vi "Open.vi"(7 "I2C Channel":u8, 8 "Error In":errorcluster, 10 "I2C Slave Address (0x1D)":u8=29 format="%.0x", 11 "LINX Ref":T1) -> (0 "Error Out":errorcluster, 3 "LINX Resource":T1)   [LabVIEW 2014, in "LMH-LINX.lvlib" / "MMA8452.lvlib"]
doc: "Open the I2C master and initialize the MMA8452 accelerometer.\n\nIf the LINX device has more than one I2C master the logical first I2C master is channel 0, the next is channel 1, etc."
uses:
  <vilib>/MakerHub/LINX/Public/Sensors/Accelerometer/MMA8452/MMA8452.lvlib
  <vilib>/MakerHub/LINX/Private/Type Defs/LINX Ref.ctl
  <vilib>/MakerHub/LINX/Private/Type Defs/Platform.ctl
  <vilib>/MakerHub/LINX/Private/Type Defs/Interface.ctl
  <vilib>/MakerHub/LINX/Private/Device/Type Defs/LINX Device Config.ctl
  <vilib>/MakerHub/LINX/Private/Device/Type Defs/TCP Config.ctl
  <vilib>/MakerHub/LINX/Private/Device/Type Defs/Channels.ctl
  <vilib>/MakerHub/LINX/Private/Type Defs/Peripherals/I2C/EOF.ctl
  <vilib>/MakerHub/LINX/Private/Local IO/LinxI2cWrite.vi
  <vilib>/MakerHub/LINX/Public/Utilities/Check Channel.vi
  <vilib>/MakerHub/LINX/Private/Utilties/Generate Error.vi
  <vilib>/MakerHub/LINX/LMH-LINX.lvlib
  <vilib>/MakerHub/LINX/Private/Device/Device.lvlib
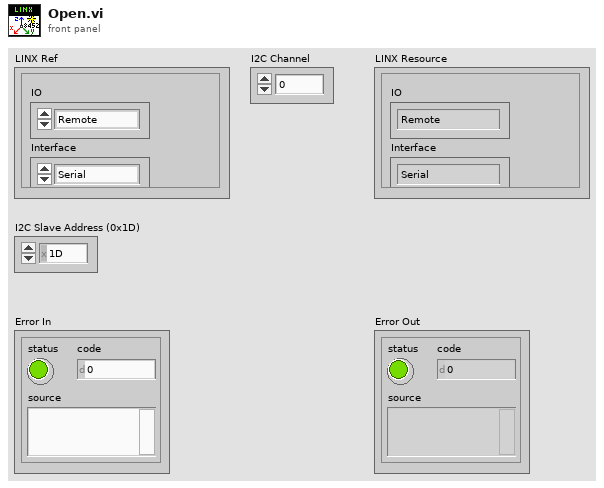
[diagram p1: front panel]
types:
  T1 = typedef "LMH-LINX.lvlib/LINX Ref.ctl" = cluster{"IO":T2, "Interface":T3, "LINX Device Config":T4}
  T2 = typedef "LMH-LINX.lvlib/Platform.ctl" = enum16{"Remote", "Local"}
  T3 = typedef "LMH-LINX.lvlib/Interface.ctl" = enum16{"Serial", "TCP"}
  T4 = typedef "LMH-LINX.lvlib/Device.lvlib/LINX Device Config.ctl" = cluster{"Interface":T3, "COM Port":refnum<visa-resource-name>, "TCP Configuration":T5, "Device Family":u8, "Device ID":u8, "Device Name":string, "TCP Ref":refnum<k5>, "Channels":T6}
  T5 = typedef "LMH-LINX.lvlib/Device.lvlib/TCP Config.ctl" = cluster{"IP Address":string, "Port":u16}
  T6 = typedef "LMH-LINX.lvlib/Channels.ctl" = cluster{"DI":u8[], "DO":u8[], "AI":u8[], "AO":u8[], "PWM":u8[], "QE":u8[], "UART":u8[], "I2C 2":u8[], "SPI":u8[], "CAN":u8[], "Servo":u8[], "AI Ref (V)":dbl, "AI Resolution (Bits)":u8, "AO Ref (V)":dbl, "AO Resolution (Bits)":u8}
  T7 = typedef "LMH-LINX.lvlib/EOF.ctl" = enum8{"Stop", "Restart", "Restart No Stop", "No Stop"}
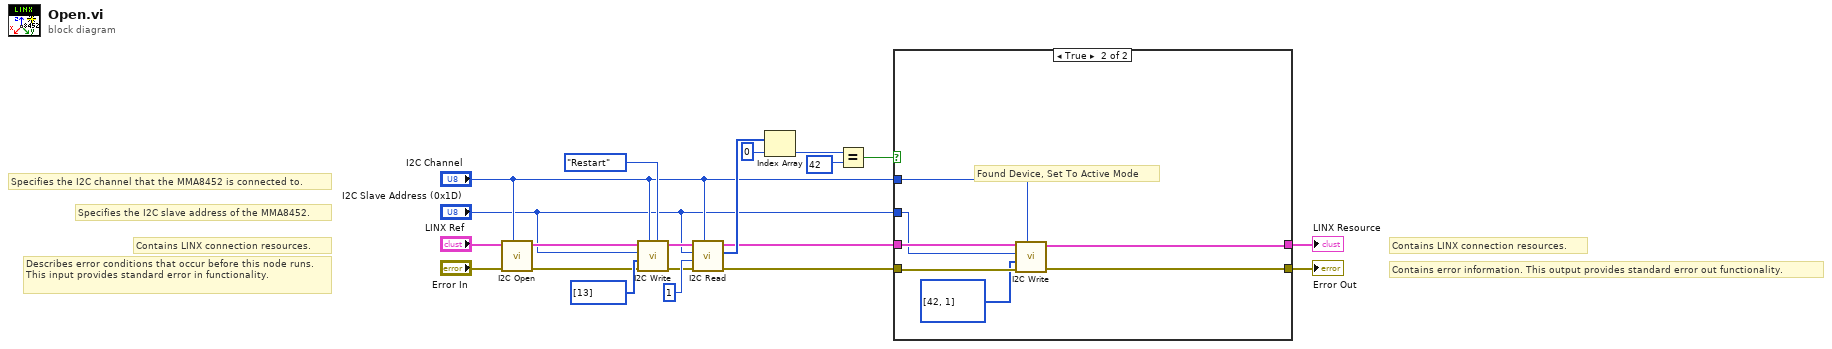
[diagram p0: block diagram]
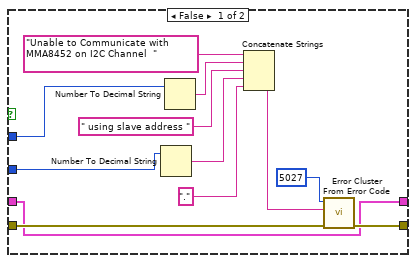
[diagram p2: hidden frame]
diagram:
  # "Contains LINX connection resources."
  # "Contains error information. This output provides standard error out functionality."
  # "Specifies the I2C slave address of the MMA8452."
  # "Specifies the I2C channel that the MMA8452 is connected to."
  # "Contains LINX connection resources."
  # "Describes error conditions that occur before this node runs. This input provides standard error in functionality."
  n1 = call <vilib>:"I2C Open.vi"("I2C Channel (0)"="I2C Channel", "Error In"="Error In", "LINX Resource"="LINX Ref") -> ("Error Out"=w11:errorcluster, "LINX Resource"=w10:T1)  [unwired: 7 in]
  n2 = call <vilib>:"I2C Write.vi"("EOF"=EOF."Restart", "I2C Channel"="I2C Channel", "Error In"=w11, "Data"=u8[] [13], "I2C Slave Address (0)"="I2C Slave Address (0x1D)", "LINX Resource"=w10) -> ("Error Out"=w14:errorcluster, "LINX Resource"=w13:T1)  [unwired: 4 in]
  n3 = call <vilib>:"I2C Read.vi"("I2C Channel"="I2C Channel", "Error In"=w14, "Bytes To Read"=u8 1, "I2C Slave Address (0)"="I2C Slave Address (0x1D)", "LINX Resource"=w13) -> ("Error Out"=w6:errorcluster, "Data"=w17:u8[], "LINX Resource"=w5:T1)  [unwired: 4 in]
  n4 = Index Array(array=w17, index=0) -> (element=w19:u8)
  n5 = Equal?(x=w19, y=u8 42) -> (x = y?=w7:bool)
  n6 = case shown="True" w7 {
    tunnel: w6 -> [w26 w36]
    tunnel: w5 -> [w21 w39]
    tunnel: [w24 w37] -> w2
    tunnel: "I2C Channel" -> [w23 w35]
    tunnel: "I2C Slave Address (0x1D)" -> [w22 w34]
    tunnel: [w21 w38] -> w1
    frame False {
      n7 = Number To Decimal String(number=w22) -> (decimal integer string=w31:string)  [unwired: 1 in]
      n8 = Number To Decimal String(number=w23) -> (decimal integer string=w29:string)  [unwired: 1 in]
      n9 = Concatenate Strings("Unable to Communicate with MMA8452 on I2C Channel  " ("error message (\"\")"), w29, " using slave address " ("string"), w31, "." ("string")) -> (w25:string)
      n10 = call <vilib>:"Error Cluster From Error Code.vi"("error in (no error)"=w26, "error message (\"\")"=w25, "error code (0)"=5027) -> ("error out"=w24:errorcluster)  [unwired: 6 in]
    }
    frame True {
      # "Found Device, Set To Active Mode"
      n11 = call <vilib>:"I2C Write.vi"("I2C Channel"=w35, "Error In"=w36, "Data"=u8[] [42, 1], "I2C Slave Address (0)"=w34, "LINX Resource"=w39) -> ("Error Out"=w37:errorcluster, "LINX Resource"=w38:T1)  [unwired: 5 in]
    }
  }
  "LINX Resource" <- w1
  "Error Out" <- w2
